vi "CommitCluster-to-MenuString.vi"(3 "Commit":T1) -> (1 "Menu String":string)   [LabVIEW 2013]
uses:
  CommitCluster.ctl
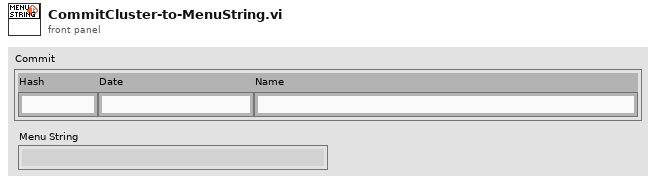
[diagram p1: front panel]
types:
  T1 = typedef "CommitCluster.ctl" = cluster{"Hash":string, "Date":string, "Name":string}
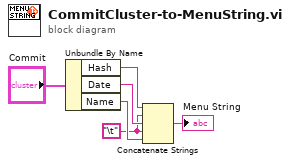
[diagram p0: block diagram]
diagram:
  w2 = "\t"
  n1 = Unbundle By Name("Commit") -> ("Hash"=w3:string, "Date"=w4:string, "Name"=w5:string)
  n2 = Concatenate Strings(w3, w2, w4, w2, w5) -> (→"Menu String":string)
